vi "VI Tree.vi"   [LabVIEW 2015, in "Zaber A Series.lvlib"]
doc: "This is the instrument driver for the Zaber ASCII Protocol. The VI Tree displays all the user-callable VIs of the instrument driver in an organized table."
uses:
  Zaber A Series.lvlib
  Action-Status/Streaming/Stream Wait for Input (Analog).vi
  Configure/Virtual Axis/Create Virtual Axis (by Angle).vi
  Action-Status/Lockstep/Lockstep Move (FW7).vi
  Action-Status/Lockstep/Lockstep Move at Velocity (FW7).vi
  Action-Status/Streaming/Set Stream Speed and Acceleration (FW7).vi
  Action-Status/Streaming/Stream Line (FW7).vi
  Action-Status/Streaming/Stream Circle (FW7).vi
  Action-Status/Streaming/Stream Arc (FW7).vi
  Action-Status/Virtual Axis/Virtual Axis Move (FW7).vi
  Action-Status/Virtual Axis/Virtual Axis Move at Velocity (FW7).vi
  Configure/Virtual Axis/Set Virtual Axis Speed (FW7).vi
  Utility/Low Level/Convert Device Units to Position Units (FW7).vi
  Utility/Low Level/Convert Device Units to Speed Units (FW7).vi
panel:
  # "(c) 2017 Zaber Technologies.  ALL RIGHTS RESERVED."
  # "SEE DIAGRAM\nFOR VI TREE."
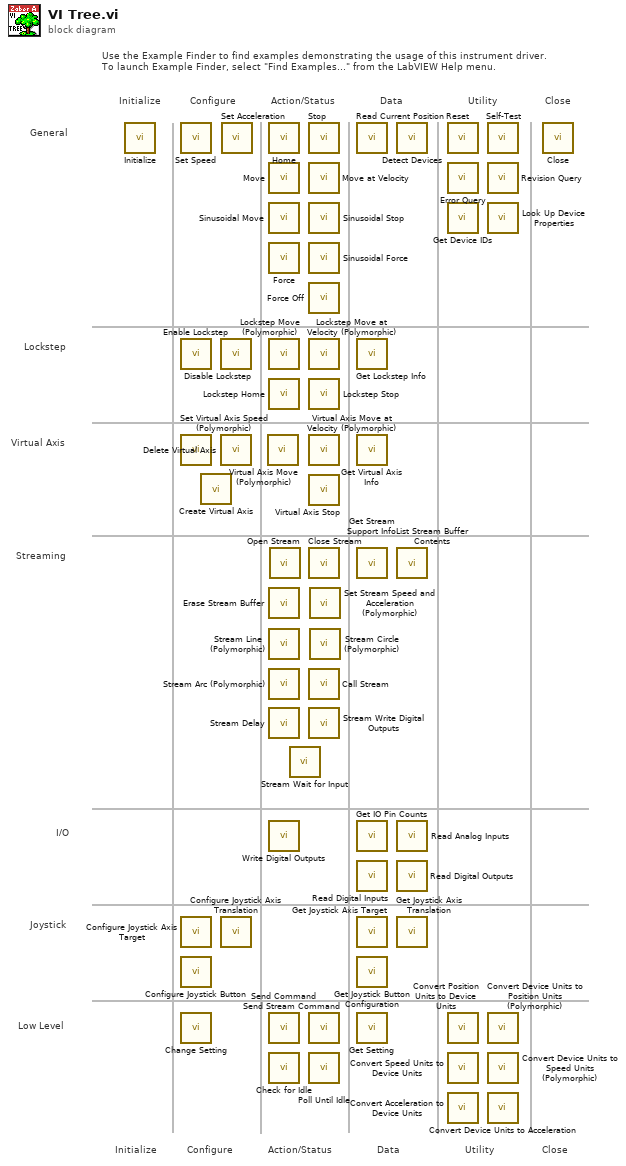
[diagram p0: block diagram]
diagram:
  # "Configure"
  # "Data"
  # "Utility"
  # "Action/Status"
  # "Close"
  # "Initialize"
  # "Joystick"
  # "Streaming"
  # "Virtual Axis"
  # "General"
  # "Lockstep"
  # "I/O"
  # "Low Level"
  # "Configure"
  # "Data"
  # "Use the Example Finder to find examples demonstrating the usage of this instrument driver.\nTo launch Example Finder, select \"Find Examples...\" from the LabVIEW Help menu."
  # "Utility"
  # "Action/Status"
  # "Close"
  # "Initialize"
  n1 = call "Initialize.vi"() -> ()  [unwired: 10 in, 2 out]
  n2 = call "Set Speed.vi"() -> ()  [unwired: 10 in, 2 out]
  n3 = call "Enable Lockstep.vi"() -> ()  [unwired: 10 in, 2 out]
  n4 = call-poly "Set Virtual Axis Speed (Polymorphic).vi"() -> ()  [unwired: 10 in, 2 out]
  n5 = call "Configure Joystick Axis Target.vi"() -> ()  [unwired: 10 in, 2 out]
  n6 = call "Configure Joystick Button.vi"() -> ()  [unwired: 10 in, 2 out]
  n7 = call "Change Setting.vi"() -> ()  [unwired: 10 in, 2 out]
  n8 = call-poly "Create Virtual Axis.vi"() -> ()  [unwired: 10 in, 2 out]
  n9 = call "Disable Lockstep.vi"() -> ()  [unwired: 10 in, 2 out]
  n10 = call "Delete Virtual Axis.vi"() -> ()  [unwired: 10 in, 2 out]
  n11 = call "Configure Joystick Axis Translation.vi"() -> ()  [unwired: 10 in, 2 out]
  n12 = call "Set Acceleration.vi"() -> ()  [unwired: 10 in, 2 out]
  n13 = call-poly "Virtual Axis Move (Polymorphic).vi"() -> ()  [unwired: 10 in, 2 out]
  n14 = call "Home.vi"() -> ()  [unwired: 10 in, 2 out]
  n15 = call "Move.vi"() -> ()  [unwired: 10 in, 2 out]
  n16 = call "Sinusoidal Move.vi"() -> ()  [unwired: 10 in, 2 out]
  n17 = call "Force.vi"() -> ()  [unwired: 10 in, 2 out]
  n18 = call-poly "Lockstep Move (Polymorphic).vi"() -> ()  [unwired: 10 in, 2 out]
  n19 = call "Lockstep Home.vi"() -> ()  [unwired: 10 in, 2 out]
  n20 = call "Erase Stream Buffer.vi"() -> ()  [unwired: 10 in, 2 out]
  n21 = call-poly "Stream Line (Polymorphic).vi"() -> ()  [unwired: 10 in, 2 out]
  n22 = call-poly "Stream Arc (Polymorphic).vi"() -> ()  [unwired: 10 in, 2 out]
  n23 = call "Stream Delay.vi"() -> ()  [unwired: 10 in, 2 out]
  n24 = call "Write Digital Outputs.vi"() -> ()  [unwired: 10 in, 2 out]
  n25 = call "Send Command.vi"() -> ()  [unwired: 6 in, 6 out]
  n26 = call "Check for Idle.vi"() -> ()  [unwired: 9 in, 3 out]
  n27 = call "Open Stream.vi"() -> ()  [unwired: 10 in, 2 out]
  n28 = call-poly "Stream Wait for Input.vi"() -> ()  [unwired: 10 in, 2 out]
  n29 = call "Stop.vi"() -> ()  [unwired: 10 in, 2 out]
  n30 = call "Move at Velocity.vi"() -> ()  [unwired: 10 in, 2 out]
  n31 = call "Sinusoidal Stop.vi"() -> ()  [unwired: 10 in, 2 out]
  n32 = call "Sinusoidal Force.vi"() -> ()  [unwired: 10 in, 2 out]
  n33 = call "Force Off.vi"() -> ()  [unwired: 10 in, 2 out]
  n34 = call-poly "Lockstep Move at Velocity (Polymorphic).vi"() -> ()  [unwired: 10 in, 2 out]
  n35 = call "Lockstep Stop.vi"() -> ()  [unwired: 10 in, 2 out]
  n36 = call-poly "Virtual Axis Move at Velocity (Polymorphic).vi"() -> ()  [unwired: 10 in, 2 out]
  n37 = call "Virtual Axis Stop.vi"() -> ()  [unwired: 10 in, 2 out]
  n38 = call "Close Stream.vi"() -> ()  [unwired: 10 in, 2 out]
  n39 = call "Call Stream.vi"() -> ()  [unwired: 10 in, 2 out]
  n40 = call "Stream Write Digital Outputs.vi"() -> ()  [unwired: 10 in, 2 out]
  n41 = call "Send Stream Command.vi"() -> ()  [unwired: 10 in, 2 out]
  n42 = call "Poll Until Idle.vi"() -> ()  [unwired: 10 in, 2 out]
  n43 = call-poly "Set Stream Speed and Acceleration (Polymorphic).vi"() -> ()  [unwired: 10 in, 2 out]
  n44 = call-poly "Stream Circle (Polymorphic).vi"() -> ()  [unwired: 10 in, 2 out]
  n45 = call "Read Current Position.vi"() -> ()  [unwired: 9 in, 3 out]
  n46 = call "Get Lockstep Info.vi"() -> ()  [unwired: 7 in, 5 out]
  n47 = call "Get Virtual Axis Info.vi"() -> ()  [unwired: 6 in, 6 out]
  n48 = call "Get Stream Support Info.vi"() -> ()  [unwired: 8 in, 4 out]
  n49 = call "Get IO Pin Counts.vi"() -> ()  [unwired: 6 in, 6 out]
  n50 = call "Read Digital Inputs.vi"() -> ()  [unwired: 9 in, 3 out]
  n51 = call "Get Joystick Axis Target.vi"() -> ()  [unwired: 7 in, 5 out]
  n52 = call "Get Joystick Button Configuration.vi"() -> ()  [unwired: 9 in, 3 out]
  n53 = call "Get Setting.vi"() -> ()  [unwired: 6 in, 6 out]
  n54 = call "Detect Devices.vi"() -> ()  [unwired: 8 in, 4 out]
  n55 = call "List Stream Buffer Contents.vi"() -> ()  [unwired: 9 in, 3 out]
  n56 = call "Read Analog Inputs.vi"() -> ()  [unwired: 9 in, 3 out]
  n57 = call "Read Digital Outputs.vi"() -> ()  [unwired: 9 in, 3 out]
  n58 = call "Get Joystick Axis Translation.vi"() -> ()  [unwired: 6 in, 6 out]
  n59 = call "Reset.vi"() -> ()  [unwired: 10 in, 2 out]
  n60 = call "Error Query.vi"() -> ()  [unwired: 8 in, 4 out]
  n61 = call "Get Device IDs.vi"() -> ()  [unwired: 8 in, 4 out]
  n62 = call "Convert Position Units to Device Units.vi"() -> ()  [unwired: 9 in, 3 out]
  n63 = call "Convert Speed Units to Device Units.vi"() -> ()  [unwired: 9 in, 3 out]
  n64 = call "Convert Acceleration to Device Units.vi"() -> ()  [unwired: 9 in, 3 out]
  n65 = call "Self-Test.vi"() -> ()  [unwired: 9 in, 3 out]
  n66 = call "Revision Query.vi"() -> ()  [unwired: 8 in, 4 out]
  n67 = call "Look Up Device Properties.vi"() -> ()  [unwired: 8 in, 4 out]
  n68 = call-poly "Convert Device Units to Position Units (Polymorphic).vi"() -> ()  [unwired: 11 in, 1 out]
  n69 = call-poly "Convert Device Units to Speed Units (Polymorphic).vi"() -> ()  [unwired: 11 in, 1 out]
  n70 = call "Convert Device Units to Acceleration.vi"() -> ()  [unwired: 11 in, 1 out]
  n71 = call "Close.vi"() -> ()  [unwired: 11 in, 1 out]
